vi "Set Values.vi"(10 "Values":refnum<class "Values.lvclass">, 11 "Processing in":refnum<class "Processing.lvclass">) -> (3 "Processing out":refnum<class "Processing.lvclass">)   [LabVIEW 2020, in "HTTP Server.lvlib" / "Processing.lvclass"]
uses:
  Processing.lvclass
  Values/Values.lvclass
  Processing.lvclass/Processing.ctl
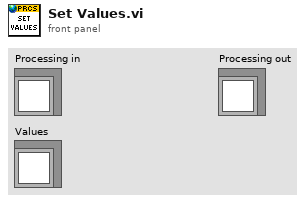
[diagram p1: front panel]
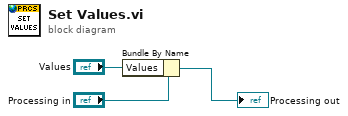
[diagram p0: block diagram]
diagram:
  n1 = Bundle By Name(cluster="Processing in", "Values"="Values") -> (→"Processing out":refnum<class "Processing.lvclass">)
